vi "New Item Progression.vi"(8 "error in (no error)":errorcluster, 9 "Progression":dbl, 10 "Status":string, 11 "Bar in":refnum<class "Bar.lvclass">) -> (0 "error out":errorcluster, 3 "Bar out":refnum<class "Bar.lvclass">)   [LabVIEW 2015, in "Simple Progress Bar.lvlib" / "Bar.lvclass"]
uses:
  Class/Bar.lvclass
  Class/Bar.lvclass/Bar.ctl
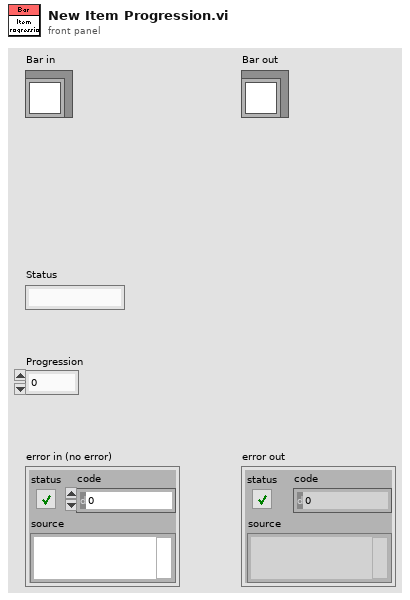
[diagram p1: front panel]
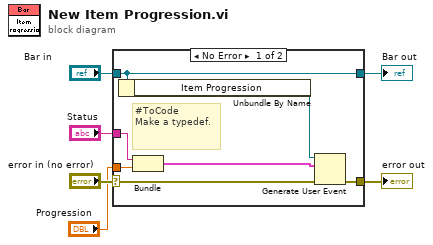
[diagram p0: block diagram]
diagram:
  n1 = case shown="No Error" "error in (no error)" {
    selector: "error in (no error)" -> [w12 w14]
    tunnel: "Bar in" -> [w10 w15]
    tunnel: [w10 w15] -> w4
    tunnel: [w11 w14] -> w3
    tunnel: "Status" -> [w8 _]
    tunnel: "Progression" -> [w7 _]
    frame No Error {
      # "#ToCode\nMake a typedef."
      n2 = Unbundle By Name(w10) -> ("Item Progression"=w13:refnum<user-event>)
      n3 = Bundle("Status"=w8, "Progression"=w7) -> (w9:cluster{"Status":string, "Progression":dbl})  [unwired: 1 in]
      n4 = Generate User Event(user event=w13, event data cluster=w9, error in=w12) -> (error out=w11:errorcluster)  [unwired: 1 in, 1 out]
    }
    frame Error {
    }
  }
  "error out" <- w3
  "Bar out" <- w4
